vi "XBee String to Queue.vi"(8 "error in (no error)":errorcluster, 10 "String Received":string, 11 "Queue cluster":T3) -> (0 "error out":errorcluster, 3 "Battery Volts":dbl)   [LabVIEW 2013]
doc: "This VI takes in the queue cluster and an XBee string, then writes that data to the correct queues.\n\nEric Schneider, April 2014"
uses:
  Data/TypeDefs/GPS-Compass Queue Cluster.ctl
  Data/TypeDefs/UTM Location.ctl
  Data/TypeDefs/WindData Queue Cluster.ctl
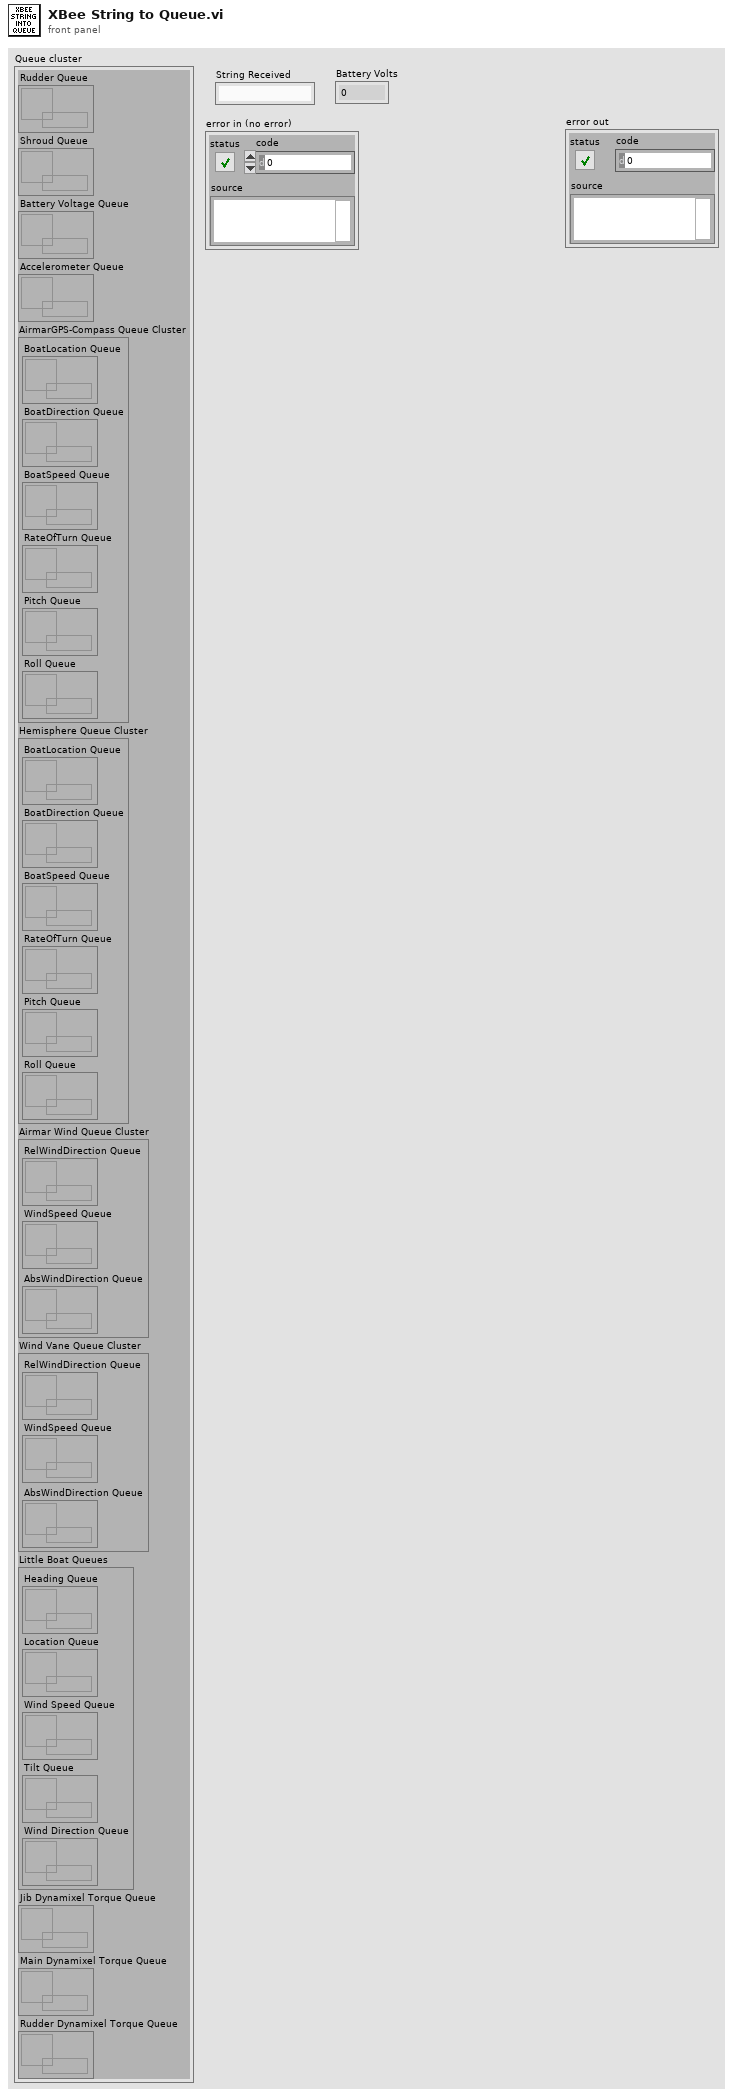
[diagram p1: front panel]
types:
  T1 = typedef "GPS-Compass Queue Cluster.ctl" = cluster{"BoatLocation Queue":refnum<queue>, "BoatDirection Queue":refnum<queue>, "BoatSpeed Queue":refnum<queue>, "RateOfTurn Queue":refnum<queue>, "Pitch Queue":refnum<queue>, "Roll Queue":refnum<queue>}
  T2 = typedef "WindData Queue Cluster.ctl" = cluster{"RelWindDirection Queue":refnum<queue>, "WindSpeed Queue":refnum<queue>, "AbsWindDirection Queue":refnum<queue>}
  T3 = cluster{"Rudder Queue":refnum<queue>, "Shroud Queue":refnum<queue>, "Battery Voltage Queue":refnum<queue>, "Accelerometer Queue":refnum<queue>, "AirmarGPS-Compass Queue Cluster":T1, "Hemisphere Queue Cluster":T1, "Airmar Wind Queue Cluster":T2, "Wind Vane Queue Cluster":T2, "Little Boat Queues":cluster{"Heading Queue":refnum<queue>, "Location Queue":refnum<queue>, "Wind Speed Queue":refnum<queue>, "Tilt Queue":refnum<queue>, "Wind Direction Queue":refnum<queue>}, "Jib Dynamixel Torque Queue":refnum<queue>, "Main Dynamixel Torque Queue":refnum<queue>, "Rudder Dynamixel Torque Queue":refnum<queue>}
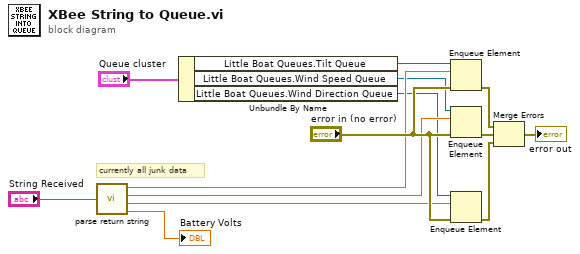
[diagram p0: block diagram]
diagram:
  # "currently all junk data"
  n1 = call "parse return string.vi"("Return String"="String Received") -> ("Tilt"=w10:dbl, "Wind Speed"=w8:dbl, "Wind Direction"=w6:dbl, "Battery Volts"=→"Battery Volts":dbl)
  n2 = Unbundle By Name("Queue cluster") -> ("Little Boat Queues.Tilt Queue"=w11:refnum<queue>, "Little Boat Queues.Wind Speed Queue"=w9:refnum<queue>, "Little Boat Queues.Wind Direction Queue"=w7:refnum<queue>)
  n3 = Enqueue Element(queue=w11, element=w10, error in (no error)="error in (no error)") -> (error out=w3:errorcluster)  [unwired: 1 in, 2 out]
  n4 = Enqueue Element(queue=w9, element=w8, error in (no error)="error in (no error)") -> (error out=w4:errorcluster)  [unwired: 1 in, 2 out]
  n5 = Enqueue Element(queue=w7, element=w6, error in (no error)="error in (no error)") -> (error out=w2:errorcluster)  [unwired: 1 in, 2 out]
  n6 = Merge Errors(w3, w4, w2) -> (→"error out":errorcluster)
